vi "JSONRPC-RetrieveMethodsInfo.vi"(11 "Method":T1(ring)) -> (3 "Output":string)   [LabVIEW 2013]
uses:
  Configuration/Global_Configurations.vi
panel:
  # "RetrieveMethodsInfo"
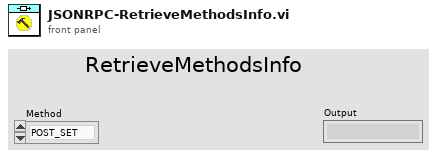
[diagram p1: front panel]
types:
  T1 = enum16{"POST_SET", "POST_GET", "SSE_GET", "GET_INFO"}
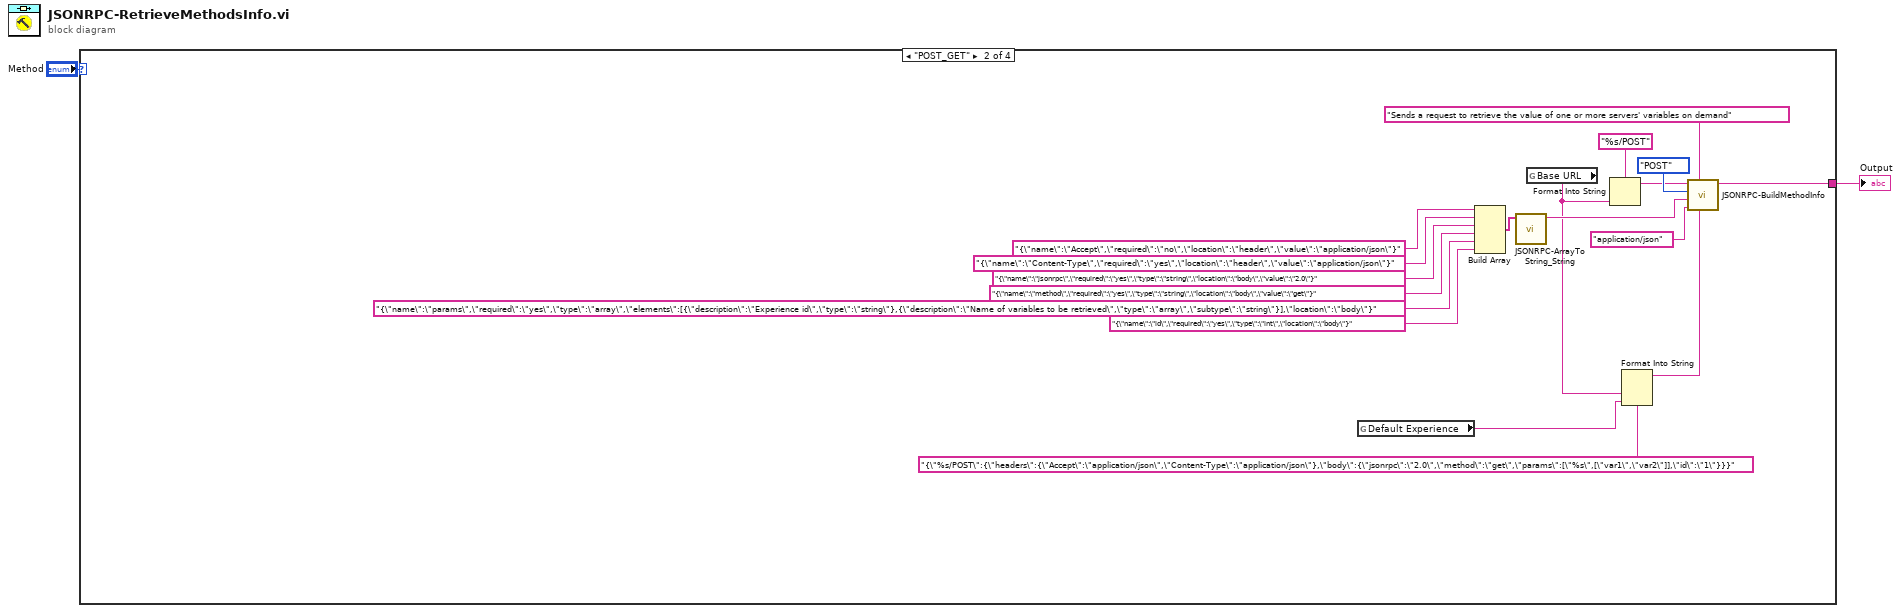
[diagram p0: block diagram]
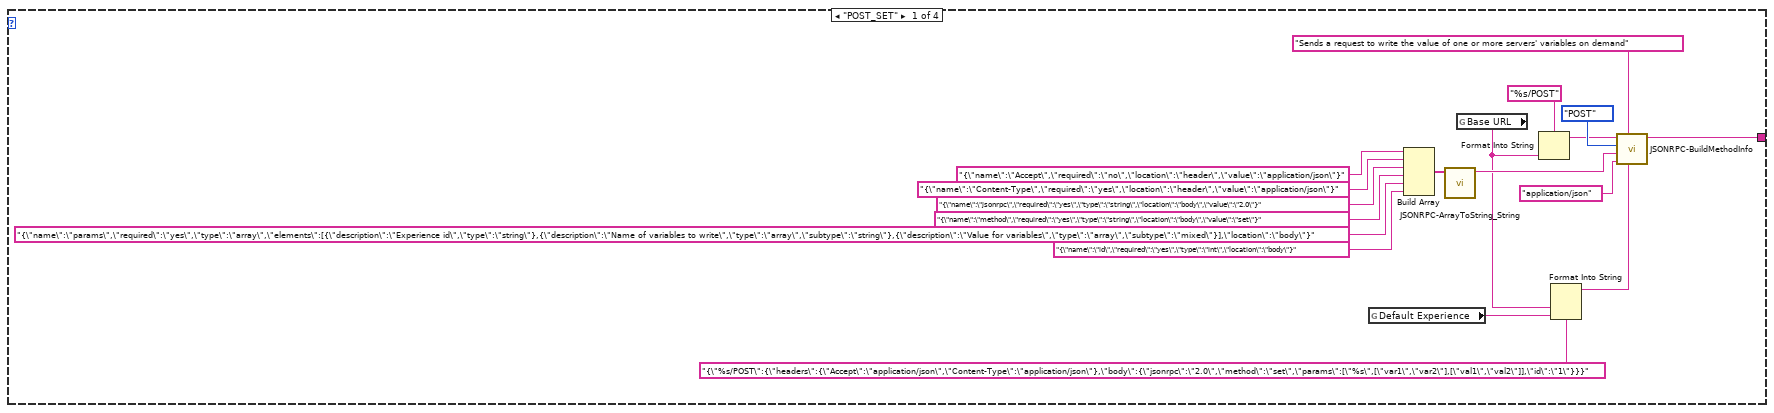
[diagram p2: hidden frame]
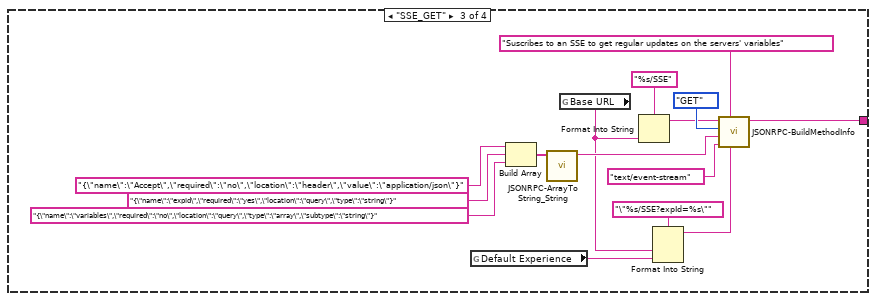
[diagram p3: hidden frame]
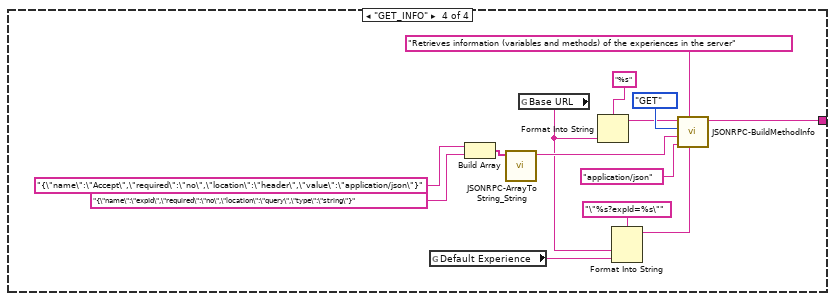
[diagram p4: hidden frame]
diagram:
  n1 = case shown="\"POST_GET\"" "Method" {
    tunnel: [w6 w24 w42 w57] -> w2
    frame "POST_SET" {
      n2 = global read "Global_Configurations.vi" "Default Experience"() -> (w20:string)
      n3 = Build Array("{\"name\":\"Accept\",\"required\":\"no\",\"location\":\"header\",\"value\":\"application/json\"}" ("Params"), "{\"name\":\"Content-Type\",\"required\":\"yes\",\"location\":\"header\",\"value\":\"application/json\"}" ("Params"), "{\"name\":\"jsonrpc\",\"required\":\"yes\",\"type\":\"string\",\"location\":\"body\",\"value\":\"2.0\"}" ("Params"), "{\"name\":\"method\",\"required\":\"yes\",\"type\":\"string\",\"location\":\"body\",\"value\":\"set\"}" ("Params"), "{\"name\":\"params\",\"required\":\"yes\",\"type\":\"array\",\"elements\":[{\"description\":\"Experience id\",\"type\":\"string\"},{\"description\":\"Name of variables to write\",\"type\":\"array\",\"subtype\":\"string\"},{\"description\":\"Value for variables\",\"type\":\"array\",\"subtype\":\"mixed\"}],\"location\":\"body\"}" ("Params"), "{\"name\":\"id\",\"required\":\"yes\",\"type\":\"int\",\"location\":\"body\"}" ("Params")) -> (w11:string[])
      n4 = call "JSONRPC-ArrayToString_String.vi"("Array"=w11) -> ("Output"=w10:string)  [unwired: 10 in]
      n5 = global read "Global_Configurations.vi" "Base URL"() -> (w4:string)
      n6 = Format Into String(format string="%s/POST", w4) -> (resulting string=w5:string)  [unwired: 2 in, 1 out]
      n7 = Format Into String(format string="{\"%s/POST\":{\"headers\":{\"Accept\":\"application/json\",\"Content-Type\":\"application/json\"},\"body\":{\"jsonrpc\":\"2.0\",\"method\":\"set\",\"params\":[\"%s\",[\"var1\",\"var2\"],[\"val1\",\"val2\"]],\"id\":\"1\"}}}", w4, w20) -> (resulting string=w19:string)  [unwired: 2 in, 1 out]
      n8 = call "JSONRPC-BuildMethodInfo.vi"("Example"=w19, "Description"="Sends a request to write the value of one or more servers' variables on demand", "Returns"="application/json", "Params"=w10, "Method"=enum16{"SSE", "GET", "POST"}."POST", "url"=w5) -> ("String"=w6:string)  [unwired: 5 in]
    }
    frame "POST_GET" {
      n9 = global read "Global_Configurations.vi" "Default Experience"() -> (w25:string)
      n10 = Build Array("{\"name\":\"Accept\",\"required\":\"no\",\"location\":\"header\",\"value\":\"application/json\"}" ("Params"), "{\"name\":\"Content-Type\",\"required\":\"yes\",\"location\":\"header\",\"value\":\"application/json\"}" ("Params"), "{\"name\":\"jsonrpc\",\"required\":\"yes\",\"type\":\"string\",\"location\":\"body\",\"value\":\"2.0\"}" ("Params"), "{\"name\":\"method\",\"required\":\"yes\",\"type\":\"string\",\"location\":\"body\",\"value\":\"get\"}" ("Params"), "{\"name\":\"params\",\"required\":\"yes\",\"type\":\"array\",\"elements\":[{\"description\":\"Experience id\",\"type\":\"string\"},{\"description\":\"Name of variables to be retrieved\",\"type\":\"array\",\"subtype\":\"string\"}],\"location\":\"body\"}" ("Params"), "{\"name\":\"id\",\"required\":\"yes\",\"type\":\"int\",\"location\":\"body\"}" ("Params")) -> (w30:string[])
      n11 = call "JSONRPC-ArrayToString_String.vi"("Array"=w30) -> ("Output"=w29:string)  [unwired: 10 in]
      n12 = global read "Global_Configurations.vi" "Base URL"() -> (w21:string)
      n13 = Format Into String(format string="%s/POST", w21) -> (resulting string=w23:string)  [unwired: 2 in, 1 out]
      n14 = Format Into String(format string="{\"%s/POST\":{\"headers\":{\"Accept\":\"application/json\",\"Content-Type\":\"application/json\"},\"body\":{\"jsonrpc\":\"2.0\",\"method\":\"get\",\"params\":[\"%s\",[\"var1\",\"var2\"]],\"id\":\"1\"}}}", w21, w25) -> (resulting string=w38:string)  [unwired: 2 in, 1 out]
      n15 = call "JSONRPC-BuildMethodInfo.vi"("Example"=w38, "Description"="Sends a request to retrieve the value of one or more servers' variables on demand", "Returns"="application/json", "Params"=w29, "Method"=enum16{"SSE", "GET", "POST"}."POST", "url"=w23) -> ("String"=w24:string)  [unwired: 5 in]
    }
    frame "SSE_GET" {
      n16 = global read "Global_Configurations.vi" "Default Experience"() -> (w53:string)
      n17 = Build Array("{\"name\":\"Accept\",\"required\":\"no\",\"location\":\"header\",\"value\":\"application/json\"}" ("Params"), "{\"name\":\"expId\",\"required\":\"yes\",\"location\":\"query\",\"type\":\"string\"}" ("Params"), "{\"name\":\"variables\",\"required\":\"no\",\"location\":\"query\",\"type\":\"array\",\"subtype\":\"string\"}" ("Params")) -> (w44:string[])
      n18 = call "JSONRPC-ArrayToString_String.vi"("Array"=w44) -> ("Output"=w43:string)  [unwired: 10 in]
      n19 = global read "Global_Configurations.vi" "Base URL"() -> (w40:string)
      n20 = Format Into String(format string="%s/SSE", w40) -> (resulting string=w39:string)  [unwired: 2 in, 1 out]
      n21 = Format Into String(format string="\"%s/SSE?expId=%s\"", w40, w53) -> (resulting string=w52:string)  [unwired: 2 in, 1 out]
      n22 = call "JSONRPC-BuildMethodInfo.vi"("Example"=w52, "Description"="Suscribes to an SSE to get regular updates on the servers' variables", "Returns"="text/event-stream", "Params"=w43, "Method"=enum16{"SSE", "GET", "POST"}."GET", "url"=w39) -> ("String"=w42:string)  [unwired: 5 in]
    }
    frame "GET_INFO" {
      n23 = global read "Global_Configurations.vi" "Default Experience"() -> (w67:string)
      n24 = Build Array("{\"name\":\"Accept\",\"required\":\"no\",\"location\":\"header\",\"value\":\"application/json\"}" ("Params"), "{\"name\":\"expId\",\"required\":\"no\",\"location\":\"query\",\"type\":\"string\"}" ("Params")) -> (w59:string[])
      n25 = call "JSONRPC-ArrayToString_String.vi"("Array"=w59) -> ("Output"=w58:string)  [unwired: 10 in]
      n26 = global read "Global_Configurations.vi" "Base URL"() -> (w55:string)
      n27 = Format Into String(format string="%s", w55) -> (resulting string=w54:string)  [unwired: 2 in, 1 out]
      n28 = Format Into String(format string="\"%s?expId=%s\"", w55, w67) -> (resulting string=w66:string)  [unwired: 2 in, 1 out]
      n29 = call "JSONRPC-BuildMethodInfo.vi"("Example"=w66, "Description"="Retrieves information (variables and methods) of the experiences in the server", "Returns"="application/json", "Params"=w58, "Method"=enum16{"SSE", "GET", "POST"}."GET", "url"=w54) -> ("String"=w57:string)  [unwired: 5 in]
    }
  }
  "Output" <- w2
